vi "TW Fix VI Missing Paths.vi"(8 "error in (no error)":errorcluster, 9 "New Subname":string, 10 "Subname to Replace":string, 11 "VI Path":path) -> (0 "error out":errorcluster)   [LabVIEW 2021]
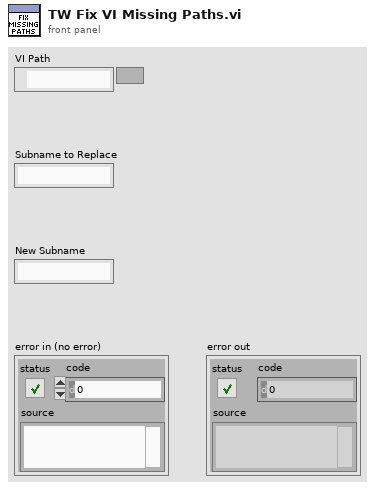
[diagram p1: front panel]
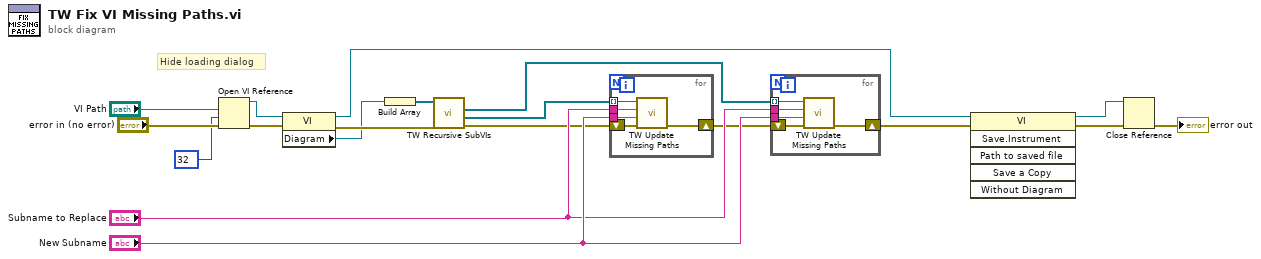
[diagram p0: block diagram]
diagram:
  # "Hide loading dialog"
  n1 = Open VI Reference(vi path="VI Path", options=32, error in (no error)="error in (no error)") -> (vi reference=w6:refnum<vi>, error out=w7:errorcluster)  [unwired: 3 in]
  n2 = property class="VI"(reference=w6, error in=w7) -> (reference out=w3:refnum<vi>, error out=w13:errorcluster, "Diagram"=w11:refnum<vi>)
  n3 = Build Array(w11) -> (w12:refnum<vi>[])
  n4 = call "TW Recursive SubVIs.vi"("error in (no error)"=w13, "Diagrams in"=w12) -> ("error out"=w15:errorcluster, "Constant references out"=w14:refnum<vi>[], "SubVI references out"=w17:refnum<vi>[])  [unwired: 7 in]
  n5 = for {
    tunnel: w14 -> [w24] mode=indexing
    shift-right: [w22] -> w16
    shift-left: w15 -> [w23]
    tunnel: "Subname to Replace" -> [w21]
    tunnel: "New Subname" -> [w20]
    n6 = call "TW Update Missing Paths.vi"("error in (no error)"=w23, "New Subname"=w20, "Subname to Replace"=w21, "GObject in"=w24) -> ("error out"=w22:errorcluster)  [unwired: 7 in]
  }
  n7 = for {
    tunnel: w17 -> [w29] mode=indexing
    shift-right: [w27] -> w4
    shift-left: w16 -> [w28]
    tunnel: "Subname to Replace" -> [w26]
    tunnel: "New Subname" -> [w25]
    n8 = call "TW Update Missing Paths.vi"("error in (no error)"=w28, "New Subname"=w25, "Subname to Replace"=w26, "GObject in"=w29) -> ("error out"=w27:errorcluster)  [unwired: 7 in]
  }
  n9 = invoke class="VI" method="Save.Instrument"(reference=w3, error in=w4) -> (reference out=w1:refnum<vi>, error out=w2:errorcluster)  [unwired: 4 in, 4 out]
  n10 = Close Reference(reference=w1, error in (no error)=w2) -> (error out=→"error out":errorcluster)
